vi "Read_register_cmd_with_page_address.vi"(7 "Words_to_read":u16, 8 "error in (no error)":errorcluster, 9 "Register Address":u8 format="%b", 10 "Page address":u8[](array[numeric]), 11 "VISA Refnum in":refnum<visa-resource-name>) -> (0 "error out":errorcluster, 3 "VISA Refnum out":refnum<visa-resource-name>, 4 "RdReg Data":u8[](array[numeric]))   [LabVIEW 2019]
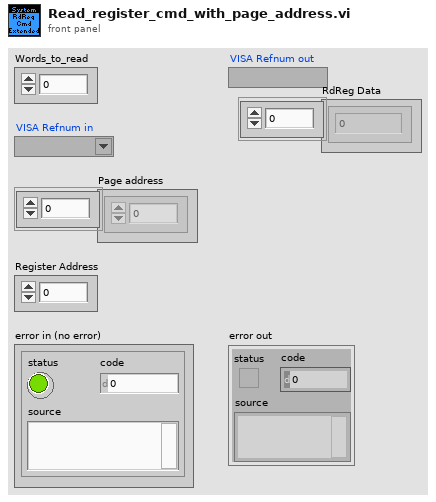
[diagram p1: front panel]
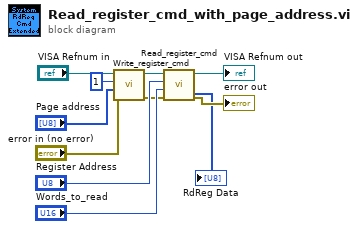
[diagram p0: block diagram]
diagram:
  n1 = call "Write_register_cmd.vi"("Arty-7 Error In"="error in (no error)", "Data Array"="Page address", "WrReg Addr"=u8 1, "Arty-7 VISA In"="VISA Refnum in") -> ("Arty-7 Error out"=w2:errorcluster, "Arty-7 VISA out"=w3:refnum<visa-resource-name>)  [unwired: 4 in, 2 out]
  n2 = call "Read_register_cmd.vi"("Arty-7 Error In"=w2, "Words_to_read"="Words_to_read", "RdReg Addr"="Register Address", "Arty-7 VISA In"=w3) -> ("Arty-7 Error out"=→"error out":errorcluster, "Arty-7 VISA out"=→"VISA Refnum out":refnum<visa-resource-name>, "RdReg Data"=→"RdReg Data":u8[])  [unwired: 3 in, 2 out]
